vi "Write D y ref.vi"(8 "error in (no error)":errorcluster, 10 "D y ref":refnum<vi>, 11 "Analyze Results Second Momentum in":refnum<class "Analyze Results Second Momentum.lvclass">) -> (0 "error out":errorcluster, 3 "Analyze Results Second Momentum out":refnum<class "Analyze Results Second Momentum.lvclass">)   [LabVIEW 2014, in "Analyze Results Second Momentum.lvclass"]
uses:
  Analyze Results Second Momentum.lvclass
  Analyze Results Second Momentum.lvclass/Analyze Results Second Momentum.ctl
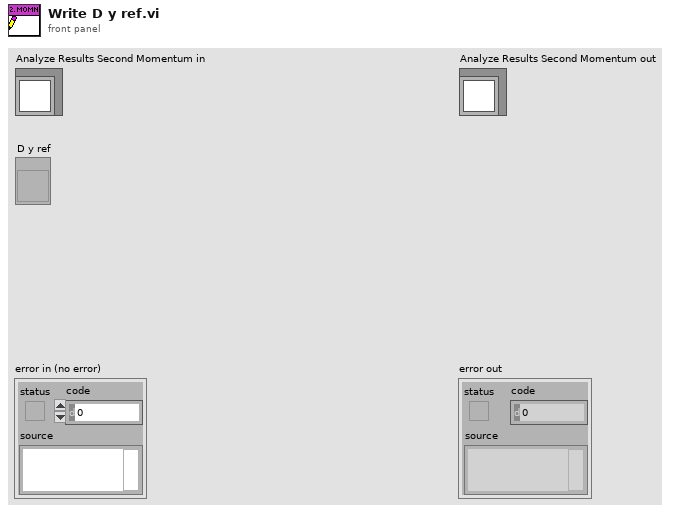
[diagram p1: front panel]
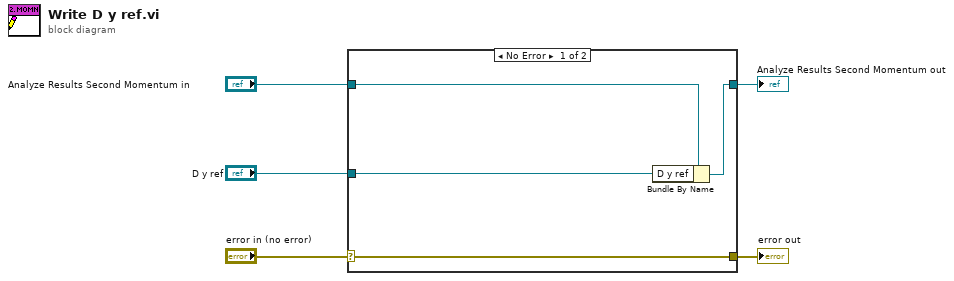
[diagram p0: block diagram]
diagram:
  n1 = case shown="No Error" "error in (no error)" {
    selector: "error in (no error)" -> [w9 w10]
    tunnel: [w9 w10] -> w4
    tunnel: [w7 w11] -> w2
    tunnel: "Analyze Results Second Momentum in" -> [w8 w11]
    tunnel: "D y ref" -> [w6 _]
    frame No Error {
      n2 = Bundle By Name(cluster=w8, "D y ref"=w6) -> (w7:refnum<class "Analyze Results Second Momentum.lvclass">)
    }
    frame Error {
    }
  }
  "error out" <- w4
  "Analyze Results Second Momentum out" <- w2
